vi "Rev Up shooter.vi"(8 "error in (no error)":errorcluster, 9 "LowSpeed":bool, 10 "MidSpeed":bool, 11 "TopSpeed":bool) -> (0 "error out":errorcluster, 2 "Speed":dbl)   [LabVIEW 2017]
uses:
  <vilib>/Rock Robotics/Network Tables/NT Read Number.vi
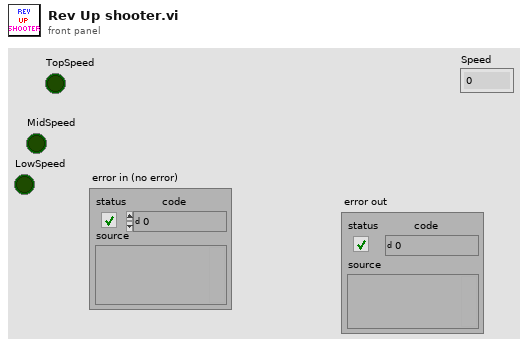
[diagram p1: front panel]
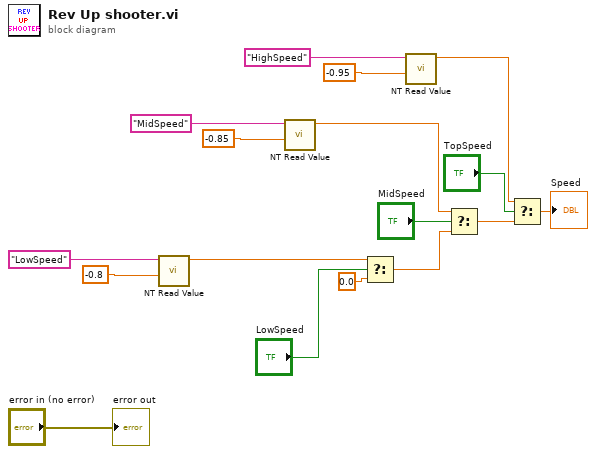
[diagram p0: block diagram]
diagram:
  n1 = call-poly <vilib>:"NT Read Value.vi"("Default Value"=-0.8, "Name"="LowSpeed") -> ("Numeric"=w1:dbl)  [unwired: 8 in, 1 out]
  n2 = call-poly <vilib>:"NT Read Value.vi"("Default Value"=-0.85, "Name"="MidSpeed") -> ("Numeric"=w6:dbl)  [unwired: 8 in, 1 out]
  n3 = Select(t=w1, s="LowSpeed", f=0.0) -> (s? t:f=w17:dbl)
  n4 = call-poly <vilib>:"NT Read Value.vi"("Default Value"=-0.95, "Name"="HighSpeed") -> ("Numeric"=w7:dbl)  [unwired: 8 in, 1 out]
  n5 = Select(t=w6, s="MidSpeed", f=w17) -> (s? t:f=w16:dbl)
  n6 = Select(t=w7, s="TopSpeed", f=w16) -> (s? t:f=→"Speed":dbl)
  "error out" <- "error in (no error)"
